vi "FIR Windowed Filter (DBL).vi"(0 "sampling freq: fs":dbl=1.0 format="%0.2f", 1 "X":dbl[](array[numeric]), 2 "filter type":T2, 3 "window parameter":dbl=nan, 7 "low cutoff freq: fl":dbl=0.125 format="%0.2f", 11 "high cutoff freq: fh":dbl=0.45 format="%0.2f", 12 "taps":i32=25 min=1, 14 "window":T1 items=["Rectangle"=0, "Hanning"=1, "Hamming"=2, "Blackman-Harris"=3, "Exact Blackman"=4, "Blackman"=5, "Flat Top"=6, "4 Term B-Harris "=7, "7 Term B-Harris"=8, "Low Sidelobe"=9, "Blackman Nuttall"=11, "Triangle"=30, "Bartlett-Hanning"=31, "Bohman"=32, "Parzen"=33, "Welch"=34, "Kaiser"=60, "Dolph-Chebyshev"=61, "Gaussian"=62]) -> (4 "Filtered X":dbl[](array[numeric]), 10 "error":i32)   [LabVIEW 2020, in "NI_AALBase.lvlib"]
doc: "Filters the input data sequence, <B>X</B>, using the set of windowed FIR filter coefficients specified by the <B>sampling freq: fs</B>, <B>low cutoff freq: fl</B>, <B>high cutoff freq: fh</B>, and number of <B>taps</B>. Wire data to the <B>X</B> input to determine the polymorphic instance to use or manually select the instance."
uses:
  <vilib>/Analysis/NI_AALBase.lvlib
  <vilib>/Analysis/3filter.llb/Filter Passband Type.ctl
  <vilib>/Analysis/4window.llb/windowTd.ctl
  <vilib>/Analysis/2dsp.llb/1D Convolution (DBL).vi
  <vilib>/Analysis/NI_AALPro.lvlib
panel:
  # "FIR Windowed Filter"
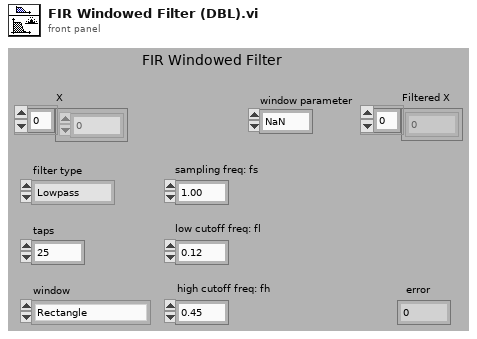
[diagram p1: front panel]
types:
  T1 = typedef "NI_AALPro.lvlib/windowTd.ctl" = u32
  T2 = typedef "NI_AALBase.lvlib/Filter Passband Type.ctl" = enum32{"Lowpass", "Highpass", "Bandpass", "Bandstop"}
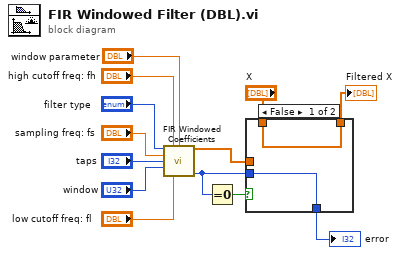
[diagram p0: block diagram]
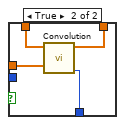
[diagram p2: hidden frame]
diagram:
  n1 = call <vilib>:"FIR Windowed Coefficients.vi"("filter type"="filter type", "high cutoff freq: fh"="high cutoff freq: fh", "window parameter"="window parameter", "sampling freq: fs"="sampling freq: fs", "taps"="taps", "window"="window", "low cutoff freq: fl"="low cutoff freq: fl") -> ("FIR Windowed Coefficients"=w9:dbl[], "error"=w2:i32)  [unwired: 1 in, 6 out]
  n2 = Equal To 0?(x=w2) -> (x = 0?=w3:bool)
  n3 = case shown="False" w3 {
    tunnel: [w15 w17] -> w12
    tunnel: w2 -> [w15 _]
    tunnel: "X" -> [w14 w19]
    tunnel: [w14 w18] -> w10
    tunnel: w9 -> [_ w16]
    frame False {
    }
    frame True {
      n4 = call-poly <vilib>:"Convolution.vi"("Y"=w16, "X"=w19) -> ("error"=w17:i32, "X * Y"=w18:dbl[])  [unwired: 1 in, 7 out]
    }
  }
  "Filtered X" <- w10
  "error" <- w12
